vi "Scenario Selection Page.vi"(8 "error in (no error)":errorcluster, 11 "Node Ptr":T1 format="%.0x") -> (0 "error out":errorcluster)   [LabVIEW 2018, in "Vires VTD System Explorer.lvlib"]
uses:
  Vires VTD System Explorer.lvlib
  <vilib>/NI Veristand/Custom Device API/Custom Device Item Ref.ctl
  <vilib>/Utility/miscctls.llb/LVRowAndColumnTypeDef.ctl
  Shared/Constants.vi
  <vilib>/NI Veristand/Custom Device API/Get Item Property (String Array).vi
  <vilib>/NI Veristand/Custom Device API/Set Item Property (String Array).vi
  <vilib>/NI Veristand/Custom Device API/Custom Device API.lvlib
  Shared/Vires VTD Shared.lvlib
panel:
  in  "Default Scenario ID":dbl
  in  "Down Arrow":bool
  in  "Up Arrow":bool
  in  "Scenario List":i32(listbox)
  in  "SHDocVw.IWebBrowser2":refnum<k7>(container)
  in  "Header":cluster{"Section Name":string}={"Section Name"="Custom Device Channel Settings"}
  in  "Description":string
  in  "Name":string
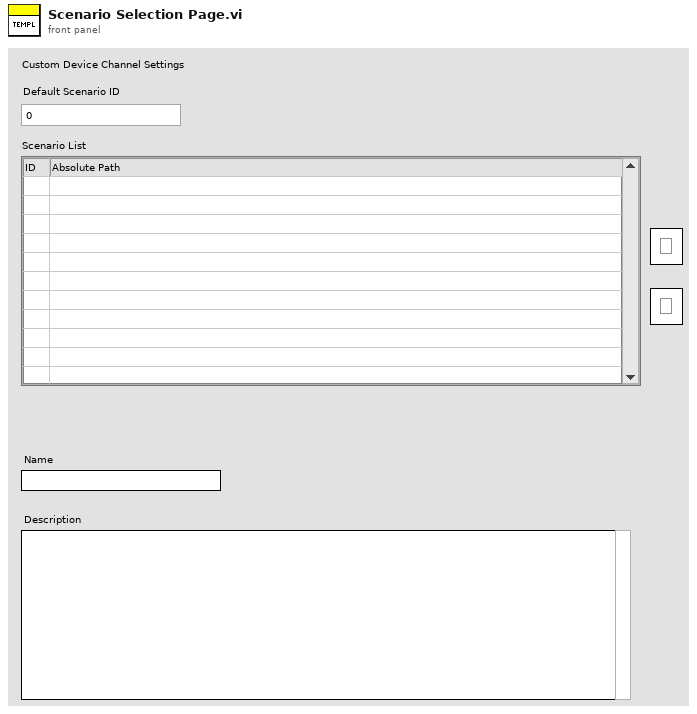
[diagram p1: front panel]
types:
  T1 = typedef "Custom Device API.lvlib/Custom Device Item Ref.ctl" = u64
  T2 = typedef "Custom Device API.lvlib/Custom Device Channel.ctl" = cluster{"Type":T3, "Units":string, "Default Value":dbl, "Faultable":bool, "Scalable":bool}
  T3 = typedef "Custom Device API.lvlib/Custom Device Channel Type.ctl" = enum16{"Input", "Output"}
  T4 = typedef "Custom Device API.lvlib/Custom Device Item Info.ctl" = cluster{"Name":string, "Is Channel":bool, "GUID":string, "Is Waveform":bool}
  T5 = typedef "LVRowAndColumnTypeDef.ctl" = cluster{"Row":i32, "Column":i32}
  T6 = typedef "Custom Device API.lvlib/Custom Device Commands.ctl" = enum16{"Default", "Item renamed", "Shutdown", "Dynamic button pressed"}
  T7 = typedef "LVPoint32TypeDef.ctl" = cluster{"Horizontal":i32, "Vertical":i32}
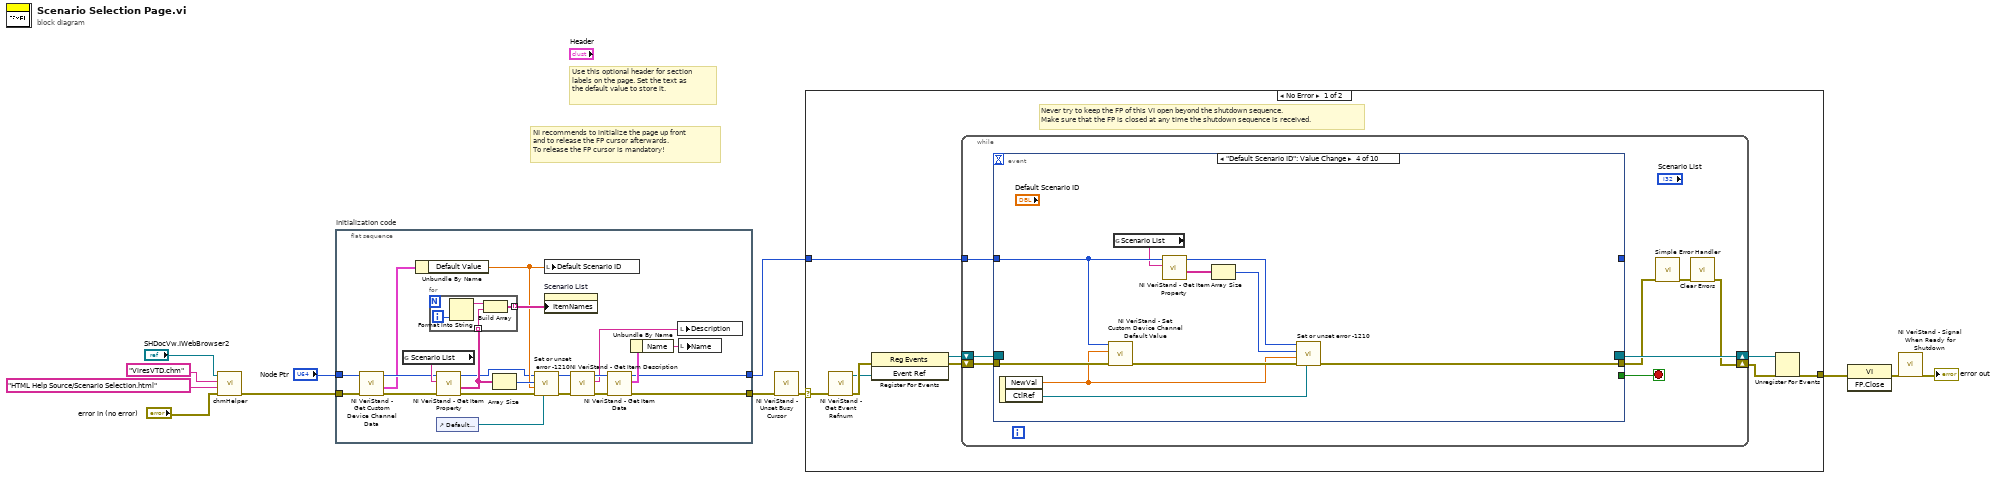
[diagram p0: block diagram]
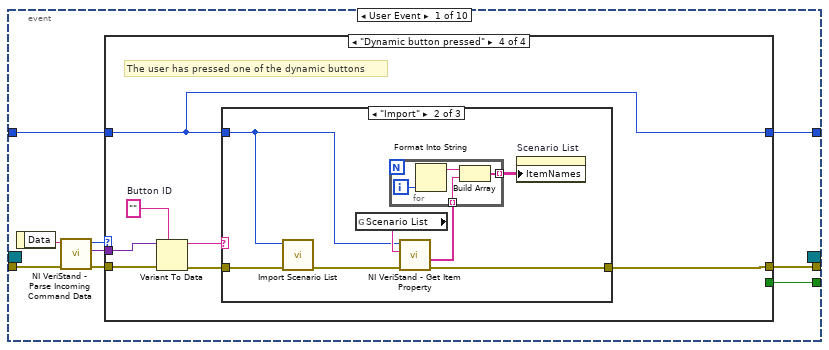
[diagram p2: hidden frame]
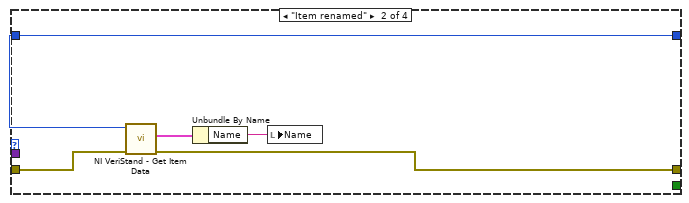
[diagram p4: hidden frame]
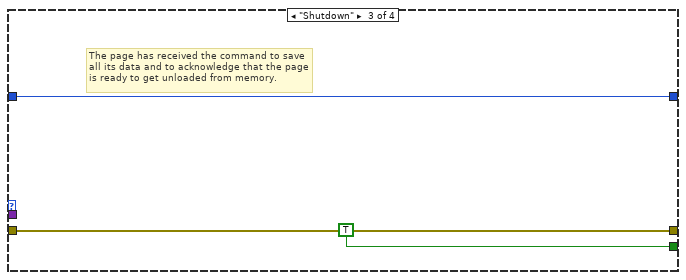
[diagram p5: hidden frame]
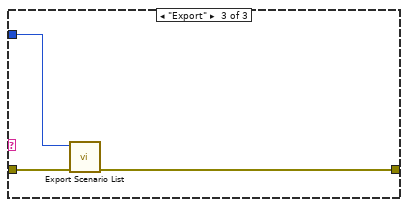
[diagram p7: hidden frame]
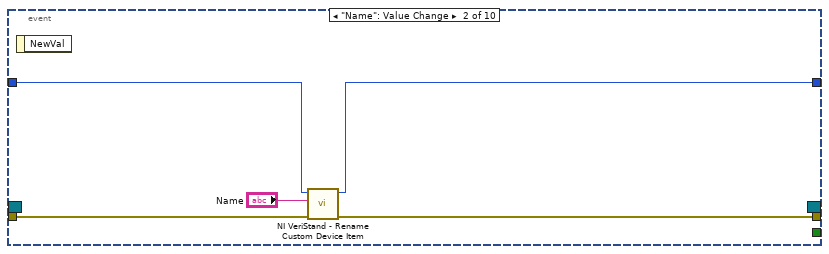
[diagram p8: hidden frame]
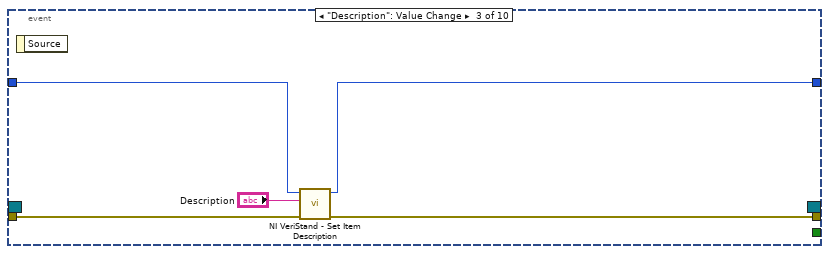
[diagram p9: hidden frame]
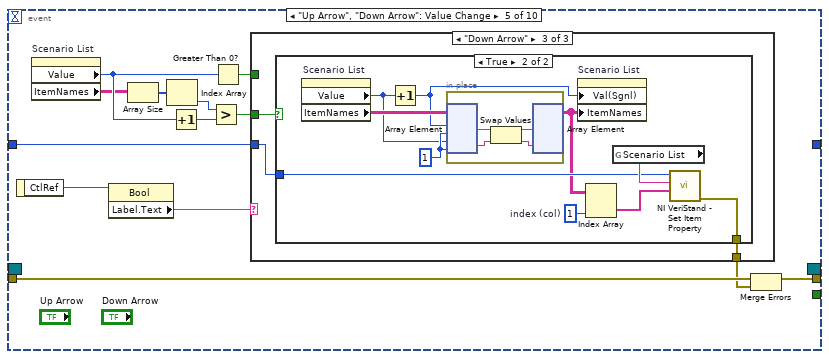
[diagram p10: hidden frame]
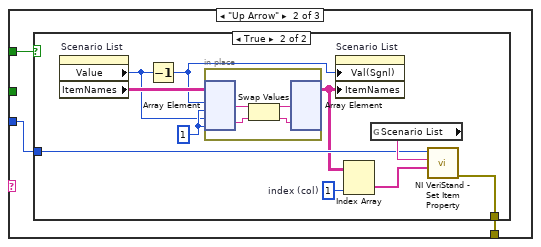
[diagram p12: hidden frame]
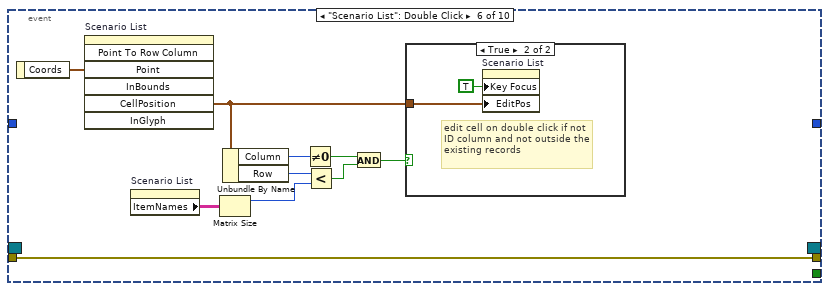
[diagram p15: hidden frame]
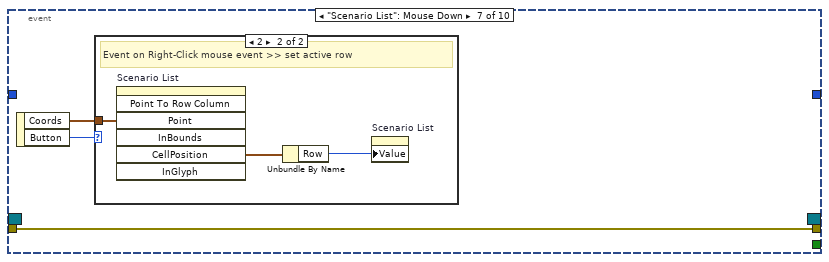
[diagram p17: hidden frame]
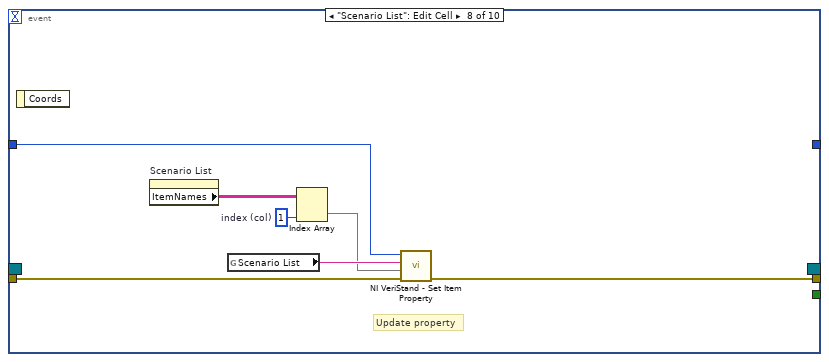
[diagram p19: hidden frame]
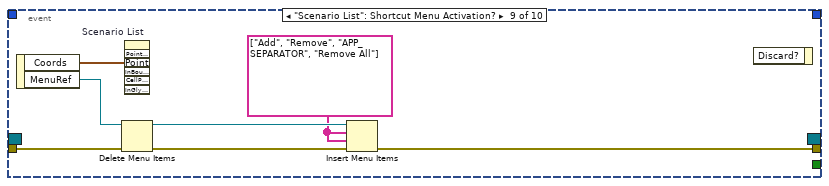
[diagram p20: hidden frame]
diagram:
  # "Use this optional header for section labels on the page. Set the text as the default value to store it."
  # "NI recommends to initialize the page up front\nand to release the FP cursor afterwards.\nTo release the FP cursor is mandatory!"
  n1 = call "chmHelper.vi"("error in (no error)"="error in (no error)", "HTML File"="HTML Help Source/Scenario Selection.html", "Main CHM File"="ViresVTD.chm" ("HTML File"), "Automation Refnum in"="SHDocVw.IWebBrowser2") -> ("error out"=w4:errorcluster)  [unwired: 7 in]
  n2 = flat-sequence "Initialization code" {
    tunnel: w4 -> [w23]
    tunnel: "Node Ptr" -> [w27]
    tunnel: [w29] -> w8
    tunnel: [w28] -> w6
    frame #0 {
      n3 = call <vilib>:"NI VeriStand - Get Custom Device Channel Data.vi"("error in (no error)"=w23, "Channel Ref in"=w27) -> ("error out"=w22:errorcluster, "Channel"=w21:T2, "Channel Ref out"=w24:T1)  [unwired: 4 in, 3 out]
      n4 = global read "Constants.vi" "Scenario List"() -> (w25:string)
      n5 = Unbundle By Name(w21) -> ("Default Value"=w19:dbl)
      n6 = call-poly <vilib>:"NI VeriStand - Get Item Property.vi"("error in (no error)"=w22, "Property Name"=w25, "Item Ref in"=w24) -> ("error out"=w15:errorcluster, "Value"=w18:string[], "Item Ref out"=w14:T1)  [unwired: 5 in, 1 out]
      n7 = for {
        tunnel: w18 -> [w36] mode=indexing
        tunnel: [w35] -> w26 mode=indexing
        i -> [w38]
        n8 = Format Into String(w38) -> (resulting string=w37:string)  [unwired: 3 in, 1 out]
        n9 = Build Array(w37, w36) -> (w35:string[])
      }
      n10 = control-ref of="Default Scenario ID"() -> (w17:refnum<vi>)
      n11 = Array Size(array=w18) -> (size(s)=w20:i32)
      n12 = call "Set or unset error -1210.vi"("ID Control Refnum"=w17, "error in"=w15, "New Default Value"=w19, "# of columns"=w20, "Item Ref In"=w14) -> ("error out"=w16:errorcluster, "Item Ref Out"=w13:T1)  [unwired: 5 in]
      n13 = local write "Default Scenario ID"(w19) -> ()
      n14 = property on="Scenario List" class="MCListbox (strict)"("ItemNames"=w26) -> ()  [unwired: 2 in, 2 out]
      n15 = call <vilib>:"NI VeriStand - Get Item Description.vi"("error in (no error)"=w16, "Item Ref in"=w13) -> ("error out"=w32:errorcluster, "Description"=w33:string, "Item Ref out"=w34:T1)  [unwired: 7 out]
      n16 = call <vilib>:"NI VeriStand - Get Item Data.vi"("error in (no error)"=w32, "Item Ref in"=w34) -> ("error out"=w29:errorcluster, "Item Info"=w31:T4, "Item Ref out"=w28:T1)  [unwired: 7 out]
      n17 = Unbundle By Name(w31) -> ("Name"=w30:string)
      n18 = local write "Description"(w33) -> ()
      n19 = local write "Name"(w30) -> ()
    }
  }
  n20 = call <vilib>:"NI VeriStand - Unset Busy Cursor.vi"("error in (no error)"=w8) -> ("error out"=w7:errorcluster)  [unwired: 10 out]
  n21 = case shown="No Error" w7 {
    selector: w7 -> [w39 w245]
    tunnel: [w44 w243] -> w12
    tunnel: w6 -> [w40 _]
    frame No Error {
      # "Never try to keep the FP of this VI open beyond the shutdown sequence.\nMake sure that the FP is closed at any time the shutdown sequence is received."
      n22 = call <vilib>:"NI VeriStand - Get Event Refnum.vi"("error in (no error)"=w39) -> ("error out"=w47:errorcluster, "Event Ref"=w43:refnum<user-event>)  [unwired: 9 out]
      n23 = register-events(error in=w47, w43) -> (reference out=w41:refnum<event-registration>, error out=w42:errorcluster)  [unwired: 1 in]
      n24 = while {
        tunnel: w40 -> [w51]
        shift-right: [w48] -> w45
        shift-left: w42 -> [w54]
        shift-right: [w55] -> w46
        shift-left: w41 -> [w53]
        stop <- w52 stop-if-true
        n25 = event shown="[3] \"Default Scenario ID\": Value Change" {
          selector: w53 -> [_ _ _ _ _ _ _ _ _ _]
          dyn-events: [_ _ _ _ _ _ _ _ _ _] -> w55
          timeout: _ -> [_ _ _ _ _ _ _ _ _ _]
          tunnel: w54 -> [w64 w101 w105 w115 w128 w169 w177 w184 w194 w197]
          tunnel: [w60 _ _ _ _ _ _ _ _ _] -> w52
          tunnel: [w59 w100 w104 w112 w118 w169 w177 w187 w189 w198] -> w50
          tunnel: w51 -> [w58 w99 w106 w109 w119 _ _ w182 _ w196]
          tunnel: [w56 w97 w102 _ _ _ _ _ _ _] -> _
          event User Event {
            n26 = event-data() -> ("Data"=w63:string)  [unwired: 1 out]
            n27 = call <vilib>:"NI VeriStand - Parse Incoming Command Data.vi"("error in (no error)"=w64, "Incoming data"=w63) -> ("error out"=w62:errorcluster, "Outgoing data"=w57:variant, "Action"=w61:T6)  [unwired: 7 out]
            n28 = case shown="\"Dynamic button pressed\"" w61 {
              tunnel: w62 -> [w66 w71 w73 w81]
              tunnel: [_ _ TRUE _] -> w60
              tunnel: [w66 w69 w73 w76] -> w59
              tunnel: w58 -> [w65 w67 w72 w78]
              tunnel: w57 -> [_ _ _ w80]
              tunnel: [w65 w67 w72 w78] -> w56
              frame "Default", Default {
              }
              frame "Item renamed" {
                n29 = call <vilib>:"NI VeriStand - Get Item Data.vi"("error in (no error)"=w71, "Item Ref in"=w67) -> ("error out"=w69:errorcluster, "Item Info"=w70:T4)  [unwired: 8 out]
                n30 = Unbundle By Name(w70) -> ("Name"=w68:string)
                n31 = local write "Name"(w68) -> ()
              }
              frame "Shutdown" {
                # "The page has received the command to save all its data and to acknowledge that the page is ready to get unloaded from memory."
              }
              frame "Dynamic button pressed" {
                w79 = ""  # Button ID
                # "The user has pressed one of the dynamic buttons"
                n32 = Variant To Data(error in=w81, type=w79, Variant=w80) -> (data=w75:string, error out=w77:errorcluster)
                n33 = case shown="\"Import\"" w75 {
                  tunnel: w78 -> [_ w83 w96]
                  tunnel: w77 -> [w82 w89 w95]
                  tunnel: [w82 w84 w94] -> w76
                  frame Default {
                  }
                  frame "Import" {
                    n34 = call "Import Scenario List.vi"("error in (no error)"=w89, "Node Ptr"=w83) -> ("error out"=w85:errorcluster)  [unwired: 9 in]
                    n35 = global read "Constants.vi" "Scenario List"() -> (w86:string)
                    n36 = call-poly <vilib>:"NI VeriStand - Get Item Property.vi"("error in (no error)"=w85, "Property Name"=w86, "Item Ref in"=w83) -> ("error out"=w84:errorcluster, "Value"=w88:string[])  [unwired: 5 in, 2 out]
                    n37 = for {
                      tunnel: w88 -> [w91] mode=indexing
                      tunnel: [w90] -> w87 mode=indexing
                      i -> [w93]
                      n38 = Format Into String(w93) -> (resulting string=w92:string)  [unwired: 3 in, 1 out]
                      n39 = Build Array(w92, w91) -> (w90:string[])
                    }
                    n40 = property on="Scenario List" class="MCListbox (strict)"("ItemNames"=w87) -> ()  [unwired: 2 in, 2 out]
                  }
                  frame "Export" {
                    n41 = call "Export Scenario List.vi"("error in (no error)"=w95, "Node Ptr"=w96) -> ("error out"=w94:errorcluster)  [unwired: 9 in]
                  }
                }
              }
            }
          }
          event "Name": Value Change {
            n42 = event-data() -> ()  [unwired: 2 out]
            n43 = call <vilib>:"NI VeriStand - Rename Custom Device Item.vi"("error in (no error)"=w101, "New Name"="Name", "Item Ref in"=w99) -> ("error out"=w100:errorcluster, "Item Ref out"=w97:T1)  [unwired: 1 in, 6 out]
          }
          event "Description": Value Change {
            n44 = event-data() -> ()  [unwired: 2 out]
            n45 = call <vilib>:"NI VeriStand - Set Item Description.vi"("error in (no error)"=w105, "Description"="Description", "Item Ref in"=w106) -> ("error out"=w104:errorcluster, "Item Ref out"=w102:T1)  [unwired: 7 out]
          }
          event "Default Scenario ID": Value Change {
            n46 = event-data() -> ("NewVal"=w111:dbl, "CtlRef"=w107:refnum<vi>)  [unwired: 1 out]
            n47 = call <vilib>:"NI VeriStand - Set Custom Device Channel Default Value.vi"("error in (no error)"=w115, "Default Value"=w111, "Channel Ref in"=w109) -> ("error out"=w113:errorcluster)  [unwired: 7 in, 1 out]
            n48 = global read "Constants.vi" "Scenario List"() -> (w108:string)
            n49 = call-poly <vilib>:"NI VeriStand - Get Item Property.vi"("Property Name"=w108, "Item Ref in"=w109) -> ("Value"=w116:string[], "Item Ref out"=w114:T1)  [unwired: 6 in, 2 out]
            n50 = Array Size(array=w116) -> (size(s)=w110:i32)
            n51 = call "Set or unset error -1210.vi"("ID Control Refnum"=w107, "error in"=w113, "New Default Value"=w111, "# of columns"=w110, "Item Ref In"=w114) -> ("error out"=w112:errorcluster)  [unwired: 5 in, 1 out]
          }
          event "Up Arrow", "Down Arrow": Value Change {
            n52 = event-data() -> ("CtlRef"=w129:refnum<vi>)  [unwired: 1 out]
            n53 = property on="Scenario List" class="MCListbox (strict)"() -> ("Value"=w126:i32, "ItemNames"=w125:string[][])  [unwired: 2 in, 2 out]
            n54 = property class="Bool"(reference=w129) -> ("Label.Text"=w127:string)  [unwired: 1 in, 2 out]
            n55 = Array Size(array=w125) -> (size(s)=w123:i32[])
            n56 = Index Array(array=w123) -> (element=w124:i32)  [unwired: 1 in]
            n57 = Increment(x=w126) -> (x+1=w122:i32)
            n58 = Greater?(x=w124, y=w122) -> (0:w121:bool)
            n59 = Greater Than 0?(x=w126) -> (x > 0?=w120:bool)
            n60 = case shown="\"Down Arrow\"" w127 {
              tunnel: w121 -> [_ _ w147]
              tunnel: w120 -> [_ w132 _]
              tunnel: w119 -> [_ w131 w149]
              tunnel: [_ w130 w148] -> w117
              frame Default {
              }
              frame "Up Arrow" {
                n61 = case shown="True" w132 {
                  tunnel: w131 -> [_ w137]
                  tunnel: [_ w136] -> w130
                  frame False {
                  }
                  frame True {
                    w134 = 1  # index (col)
                    w142 = 1
                    n62 = property on="Scenario List" class="MCListbox (strict)"() -> ("Value"=w139:i32, "ItemNames"=w141:string[][])  [unwired: 2 in, 2 out]
                    n63 = Decrement(x=w139) -> (x-1=w140:i32)
                    n64 = in-place {
                      n65 = in-place-array #1(w141, w140, w142, w139, w142) -> (w146:string, w145:string)
                      n66 = Swap Values(12:w146, 14:w145) -> (1:w144:string, 3:w143:string)  [unwired: 1 out]
                      n67 = in-place-array #1(w144, w143) -> (w135:string[][])  [unwired: 4 out]
                    }
                    n68 = property on="Scenario List" class="MCListbox (strict)"("Val(Sgnl)"=w140, "ItemNames"=w135) -> ()  [unwired: 2 in, 2 out]
                    n69 = Index Array(array=w135, index (col)=w134) -> (element=w133:string[])  [unwired: 1 in]
                    n70 = global read "Constants.vi" "Scenario List"() -> (w138:string)
                    n71 = call-poly <vilib>:"NI VeriStand - Set Item Property.vi"("Value"=w133, "Property Name"=w138, "Item Ref in"=w137) -> ("error out"=w136:errorcluster)  [unwired: 6 in, 2 out]
                  }
                }
              }
              frame "Down Arrow" {
                n72 = case shown="True" w147 {
                  tunnel: w149 -> [_ w154]
                  tunnel: [_ w153] -> w148
                  frame False {
                  }
                  frame True {
                    w151 = 1  # index (col)
                    w159 = 1
                    n73 = property on="Scenario List" class="MCListbox (strict)"() -> ("Value"=w156:i32, "ItemNames"=w158:string[][])  [unwired: 2 in, 2 out]
                    n74 = Increment(x=w156) -> (x+1=w157:i32)
                    n75 = in-place {
                      n76 = in-place-array #2(w158, w157, w159, w156, w159) -> (w163:string, w162:string)
                      n77 = Swap Values(12:w163, 14:w162) -> (1:w161:string, 3:w160:string)  [unwired: 1 out]
                      n78 = in-place-array #2(w161, w160) -> (w152:string[][])  [unwired: 4 out]
                    }
                    n79 = property on="Scenario List" class="MCListbox (strict)"("Val(Sgnl)"=w157, "ItemNames"=w152) -> ()  [unwired: 2 in, 2 out]
                    n80 = Index Array(array=w152, index (col)=w151) -> (element=w150:string[])  [unwired: 1 in]
                    n81 = global read "Constants.vi" "Scenario List"() -> (w155:string)
                    n82 = call-poly <vilib>:"NI VeriStand - Set Item Property.vi"("Value"=w150, "Property Name"=w155, "Item Ref in"=w154) -> ("error out"=w153:errorcluster)  [unwired: 6 in, 2 out]
                  }
                }
              }
            }
            n83 = Merge Errors(w128, w117) -> (w118:errorcluster)
          }
          event "Scenario List": Double Click {
            n84 = event-data() -> ("Coords"=w173:T7)  [unwired: 1 out]
            n85 = invoke on="Scenario List" class="MCListbox (strict)" method="Point To Row Column"("Point"=w173) -> ("CellPosition"=w172:T5)  [unwired: 6 in, 6 out]
            n86 = property on="Scenario List" class="MCListbox (strict)"() -> ("ItemNames"=w165:string[][])  [unwired: 2 in, 2 out]
            n87 = Matrix Size(0:w165) -> (1:w164:i32)  [unwired: 1 out]
            n88 = Unbundle By Name(w172) -> ("Column"=w171:i32, "Row"=w168:i32)
            n89 = Not Equal To 0?(x=w171) -> (x != 0?=w170:bool)
            n90 = Less?(x=w168, y=w164) -> (x < y?=w167:bool)
            n91 = And(x=w170, y=w167) -> (x .and. y?=w166:bool)
            n92 = case shown="True" w166 {
              tunnel: w172 -> [_ w175]
              frame False {
              }
              frame True {
                # "edit cell on double click if not ID column and not outside the existing records"
                n93 = property on="Scenario List" class="MCListbox (strict)"("Key Focus"=TRUE, "EditPos"=w175) -> ()  [unwired: 2 in, 2 out]
              }
            }
          }
          event "Scenario List": Mouse Down {
            n94 = event-data() -> ("Coords"=w178:T7, "Button"=w176:u16)  [unwired: 1 out]
            n95 = case shown="2" w176 {
              tunnel: w178 -> [_ w181]
              frame 0, Default {
              }
              frame 2 {
                # "Event on Right-Click mouse event >> set active row"
                n96 = invoke on="Scenario List" class="MCListbox (strict)" method="Point To Row Column"("Point"=w181) -> ("CellPosition"=w180:T5)  [unwired: 6 in, 6 out]
                n97 = Unbundle By Name(w180) -> ("Row"=w179:i32)
                n98 = property on="Scenario List" class="MCListbox (strict)"("Value"=w179) -> ()  [unwired: 2 in, 2 out]
              }
            }
          }
          event "Scenario List": Edit Cell {
            w186 = 1  # index (col)
            # "Update property"
            n99 = event-data() -> ()  [unwired: 2 out]
            n100 = property on="Scenario List" class="MCListbox (strict)"() -> ("ItemNames"=w183:string[][])  [unwired: 2 in, 2 out]
            n101 = global read "Constants.vi" "Scenario List"() -> (w188:string)
            n102 = Index Array(array=w183, index (col)=w186) -> (element=w185:string[])  [unwired: 1 in]
            n103 = call-poly <vilib>:"NI VeriStand - Set Item Property.vi"("error in (no error)"=w184, "Value"=w185, "Property Name"=w188, "Item Ref in"=w182) -> ("error out"=w187:errorcluster)  [unwired: 5 in, 2 out]
          }
          event "Scenario List": Shortcut Menu Activation? {
            w190 = string[] ["Add", "Remove", "APP_SEPARATOR", "Remove All"] ("item names")
            n104 = event-data() -> ("Coords"=w193:T7, "MenuRef"=w195:refnum<k9>)  [unwired: 1 out]
            n105 = Delete Menu Items(6:w194, 9:w195) -> (0:w192:errorcluster, 3:w191:refnum<k9>)  [unwired: 2 in]
            n106 = invoke on="Scenario List" class="MCListbox (strict)" method="Point To Row Column"("Point"=w193) -> ()  [unwired: 6 in, 7 out]
            n107 = Insert Menu Items(6:w192, 7:w190, 8:w190, 9:w191) -> (0:w189:errorcluster)  [unwired: 2 in, 2 out]
            n108 = event-data() -> ()  [unwired: 2 in, 1 out]
          }
          event "Scenario List": Shortcut Menu Selection (User) {
            n109 = event-data() -> ("CtlRef"=w201:refnum<vi>, "Coords"=w202:T7, "ItemTag"=w200:string)  [unwired: 1 out]
            n110 = invoke on="Invoke Node" class="MCListbox (strict)" method="Point To Row Column"(reference=w201, "Point"=w202) -> ("CellPosition"=w199:T5)  [unwired: 5 in, 6 out]
            n111 = case shown="\"Remove\"" w200 {
              tunnel: w199 -> [w210 _ _ _]
              tunnel: [w207 w224 w231 w242] -> w198
              tunnel: w197 -> [w205 w223 w231 w242]
              tunnel: w196 -> [w204 w222 _ _]
              frame "Remove" {
                w212 = 1  # disabled index (col)
                # "Trigger coersion of default ID"
                n112 = Unbundle By Name(w210) -> ("Row"=w209:i32)
                n113 = property on="Scenario List" class="MCListbox (strict)"() -> ("ItemNames"=w213:string[][])  [unwired: 2 in, 2 out]
                n114 = Index Array(array=w213, index (col)=w212) -> (element=w211:string[])  [unwired: 1 in]
                n115 = Delete From Array(array=w211, index=w209) -> (array with subset deleted=w206:string[])  [unwired: 1 in, 1 out]
                n116 = for {
                  tunnel: [w216] -> w214 mode=indexing
                  tunnel: w206 -> [w215] mode=indexing
                  i -> [w218]
                  n117 = Format Into String(w218) -> (resulting string=w217:string)  [unwired: 3 in, 1 out]
                  n118 = Build Array(w217, w215) -> (w216:string[])
                }
                n119 = global read "Constants.vi" "Scenario List"() -> (w208:string)
                n120 = property on="Scenario List" class="MCListbox (strict)"("ItemNames"=w214) -> ()  [unwired: 2 in, 2 out]
                n121 = call-poly <vilib>:"NI VeriStand - Set Item Property.vi"("error in (no error)"=w205, "Value"=w206, "Property Name"=w208, "Item Ref in"=w204) -> ("error out"=w207:errorcluster)  [unwired: 5 in, 2 out]
                n122 = local read "Default Scenario ID"() -> (w203:dbl)
                n123 = property on="Default Scenario ID" class="DigNum (strict)"("Val(Sgnl)"=w203) -> ()  [unwired: 2 in, 2 out]
              }
              frame "Remove All" {
                w220 = string[] []  # Empty
                # "Trigger coersion of default ID"
                n124 = Build Array(w220) -> (w221:string[][])
                n125 = global read "Constants.vi" "Scenario List"() -> (w225:string)
                n126 = property on="Scenario List" class="MCListbox (strict)"("ItemNames"=w221) -> ()  [unwired: 2 in, 2 out]
                n127 = call-poly <vilib>:"NI VeriStand - Set Item Property.vi"("error in (no error)"=w223, "Value"=w220, "Property Name"=w225, "Item Ref in"=w222) -> ("error out"=w224:errorcluster)  [unwired: 5 in, 2 out]
                n128 = property on="Default Scenario ID" class="DigNum (strict)"("Val(Sgnl)"=0.0 ("Value (Signaling)")) -> ()  [unwired: 2 in, 2 out]
              }
              frame "Add" {
                w236 = 1  # disabled index (col)
                n129 = property on="Scenario List" class="MCListbox (strict)"() -> ("ItemNames"=w237:string[][])  [unwired: 2 in, 2 out]
                n130 = Index Array(array=w237, index (col)=w236) -> (element=w234:string[])  [unwired: 1 in]
                n131 = Build Array (concatenate)(w234, "<path to scenario>") -> (w230:string[])
                n132 = for {
                  tunnel: [w240] -> w232 mode=indexing
                  tunnel: w230 -> [w239] mode=indexing
                  i -> [w238]
                  n133 = Format Into String(w238) -> (resulting string=w241:string)  [unwired: 3 in, 1 out]
                  n134 = Build Array(w241, w239) -> (w240:string[])
                }
                n135 = Array Size(array=w230) -> (size(s)=w229:i32)
                n136 = Decrement(x=w229) -> (x-1=w228:i32)
                n137 = Bundle(cluster=T5 {"Row"=0, "Column"=1} ("Edit Position"), "Row"=w228) -> (w227:T5)  [unwired: 1 in]
                n138 = property on="Scenario List" class="MCListbox (strict)"("ItemNames"=w232, "Value"=w228, "Key Focus"=TRUE, "EditPos"=w227) -> ()  [unwired: 2 in, 2 out]
              }
              frame Default {
              }
            }
          }
        }
        n139 = call <vilib>:"Simple Error Handler.vi"("error in (no error)"=w50) -> ("error out"=w49:errorcluster)  [unwired: 1 in, 7 out]
        n140 = call <vilib>:"Clear Errors.vi"("error in (no error)"=w49) -> ("error out"=w48:errorcluster)  [unwired: 1 in, 5 out]
      }
      n141 = Unregister For Events(event registration refnum=w46, error in=w45) -> (error out=w44:errorcluster)
    }
    frame Error {
      n142 = call <vilib>:"Simple Error Handler.vi"("error in (no error)"=w245) -> ("error out"=w244:errorcluster)  [unwired: 1 in, 7 out]
      n143 = call <vilib>:"Clear Errors.vi"("error in (no error)"=w244) -> ("error out"=w243:errorcluster)  [unwired: 1 in, 5 out]
    }
  }
  n144 = invoke class="VI" method="FP.Close"(error in=w12) -> (error out=w11:errorcluster)  [unwired: 2 in, 2 out]
  n145 = call <vilib>:"NI VeriStand - Signal When Ready for Shutdown.vi"("error in (no error)"=w11) -> ("error out"=→"error out":errorcluster)  [unwired: 10 out]
